vi "Preview Elements.vi"(8 "error in":errorcluster, 9 "count (-1: all)":i32=-1, 11 "ByteBuffer in":refnum<data-value>) -> (0 "error out":errorcluster, 2 "elements":variant[](array[variant]), 3 "ByteBuffer":refnum<data-value>)   [LabVIEW 2013, in "VariantBuffer.lvclass"]
doc: "This VI returns data from the ring buffer starting from the oldest data and ending with the newest.\n\nThe data is duplicated at the output so this VI allocates new place in the memory for the output."
uses:
  VariantBuffer.lvclass
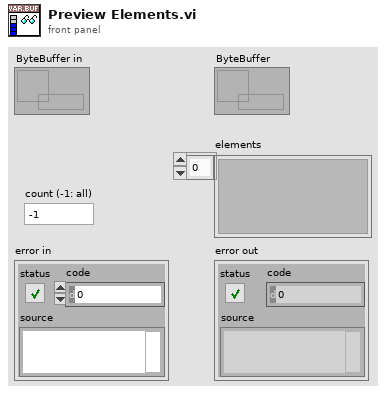
[diagram p1: front panel]
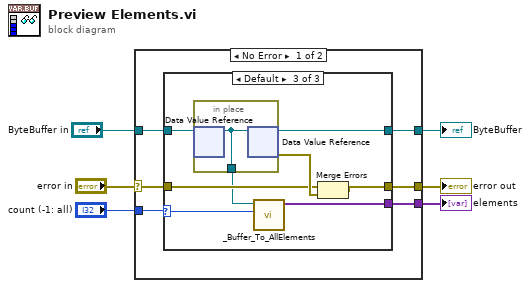
[diagram p0: block diagram]
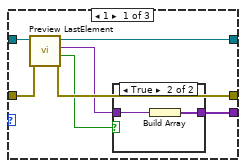
[diagram p2: hidden frame]
diagram:
  n1 = case shown="No Error" "error in" {
    selector: "error in" -> [w8 w33]
    tunnel: "ByteBuffer in" -> [w12 w34]
    tunnel: [w11 w34] -> w5
    tunnel: [w10 w33] -> w2
    tunnel: [w9 _] -> w4
    tunnel: "count (-1: all)" -> [w7 _]
    frame No Error {
      n2 = case shown="Default" w7 {
        selector: w7 -> [_ _ w26]
        tunnel: w12 -> [w19 w23 w31]
        tunnel: [w18 w23 w30] -> w11
        tunnel: [w16 w22 w28] -> w10
        tunnel: [w14 _ w25] -> w9
        tunnel: w8 -> [w17 w22 w27]
        frame 1 {
          n3 = call "Preview LastElement.vi"("error in"=w17, "Buffer in"=w19) -> ("error out"=w16:errorcluster, "found"=w13:bool, "element"=w15:variant, "Buffer"=w18:refnum<data-value>)  [unwired: 6 in]
          n4 = case shown="True" w13 {
            tunnel: w15 -> [_ w21]
            tunnel: [_ w20] -> w14
            frame False {
            }
            frame True {
              n5 = Build Array(w21) -> (w20:variant[])
            }
          }
        }
        frame 0 {
        }
        frame Default {
          n6 = in-place {
            in-place-border: [w32] -> w24
            n7 = in-place-dvr #1(w31) -> (w32:refnum<class "VariantBuffer.lvclass">)  [unwired: 1 out]
            n8 = in-place-dvr #1(w32) -> (w30:refnum<data-value>, w29:errorcluster)
          }
          n9 = call "_Buffer_To_AllElements.vi"("count (-1: all)"=w26, "Buffer"=w24) -> ("elements"=w25:variant[])  [unwired: 9 in]
          n10 = Merge Errors(w27, w29) -> (w28:errorcluster)
        }
      }
    }
    frame Error {
    }
  }
  "error out" <- w2
  "ByteBuffer" <- w5
  "elements" <- w4
